vi "1 Stable Data Reader.vi"(8 "error in":errorcluster, 11 "VISA resource name":refnum<visa-resource-name>) -> (0 "error out":errorcluster, 1 "Stable":bool, 2 "Weight":dbl format="%.2f", 3 "VISA resource name out":refnum<visa-resource-name>, 4 "read buffer":string, 5 "Unit":string)   [LabVIEW 2014, in "AD4212C.lvlib"]
uses:
  AD4212C.lvlib
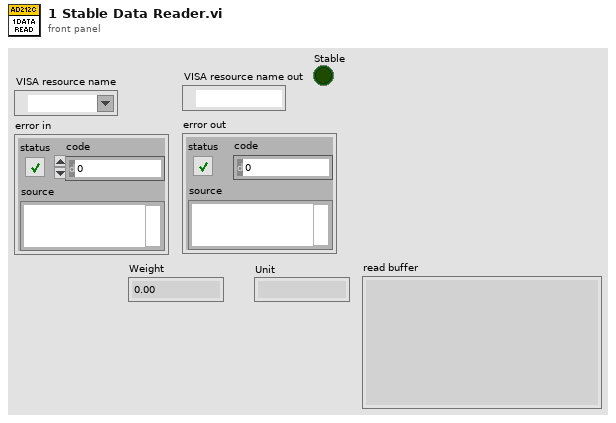
[diagram p1: front panel]
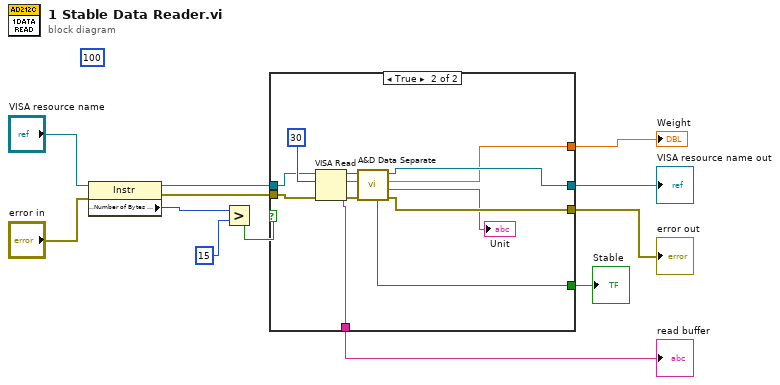
[diagram p0: block diagram]
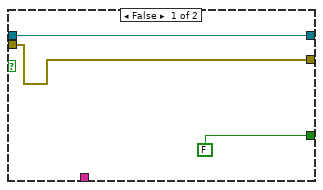
[diagram p2: hidden frame]
diagram:
  (unwired) 100
  n1 = property class="Instr"(reference="VISA resource name", error in="error in") -> (reference out=w4:refnum<visa-resource-name>, error out=w3:errorcluster, "Serial Settings:Number of Bytes at Serial Port"=w6:u32)
  n2 = Greater?(x=w6, y=u32 15) -> (0:w5:bool)
  n3 = case shown="True" w5 {
    tunnel: w4 -> [w15 w25]
    tunnel: w3 -> [w14 w24]
    tunnel: [w15 w19] -> w9
    tunnel: [w14 w21] -> w8
    tunnel: [_ w18] -> w10
    tunnel: [FALSE ("Stable") w17] -> w2
    tunnel: [_ w16] -> w1
    frame False {
    }
    frame True {
      n4 = VISA Read(VISA resource name=w25, byte count=u32 30 ("バイトカウント（0）"), error in (no error)=w24) -> (VISA resource name out=w23:refnum<visa-resource-name>, read buffer=w16:string, error out=w22:errorcluster)  [unwired: 1 out]
      n5 = call "A&D Data Separate.vi"("error in (no error)"=w22, "Received Data"=w16, "VISA resource name"=w23) -> ("error out"=w21:errorcluster, "Unit"=→"Unit":string, "Value"=w18:dbl, "VISA resource name out"=w19:refnum<visa-resource-name>, "Stable"=w17:bool)  [unwired: 4 in]
    }
  }
  "Weight" <- w10
  "VISA resource name out" <- w9
  "error out" <- w8
  "Stable" <- w2
  "read buffer" <- w1
